vi "step6 Solve.vi"(8 "error in (no error)":errorcluster, 11 "cube in":T1) -> (0 "error out":errorcluster, 1 "all corners solved?":bool, 3 "cube out":T1)   [LabVIEW 2011]
doc: "Rotate cube as necessary so that the top middle piece matches the desired start colour.\n\nNo transformations are done in this VI, the operations are loaded on the the operation queue bus."
uses:
  Typedef/cube.ctl
  Typedef/face.ctl
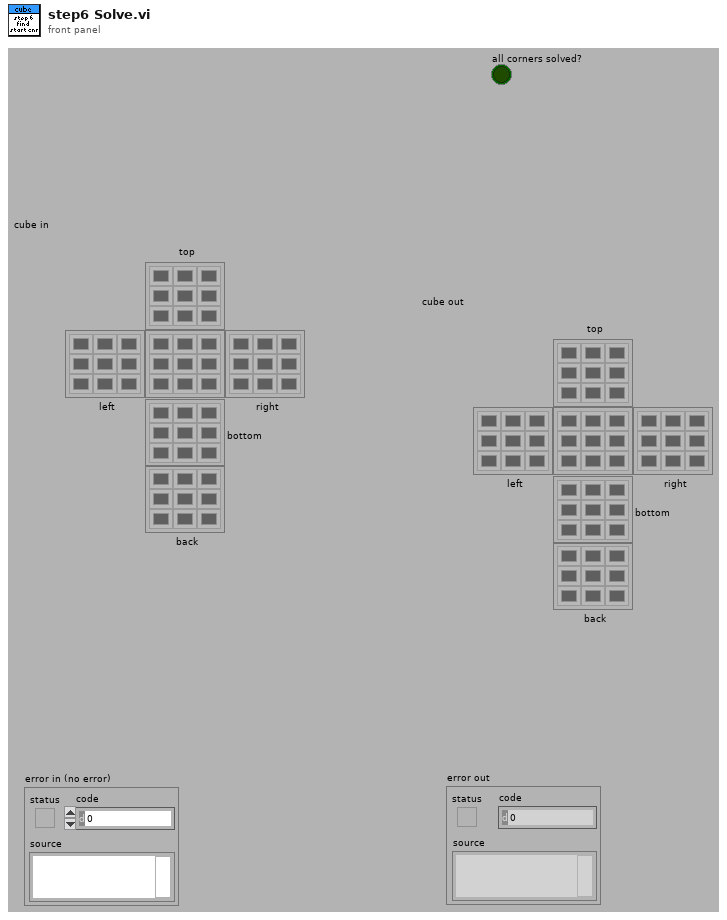
[diagram p1: front panel]
types:
  T1 = typedef "cube.ctl" = cluster{"top":T2, "left":T2, "right":T2, "bottom":T2, "back":T2, "front":T2}
  T2 = typedef "face.ctl" = u32[][]
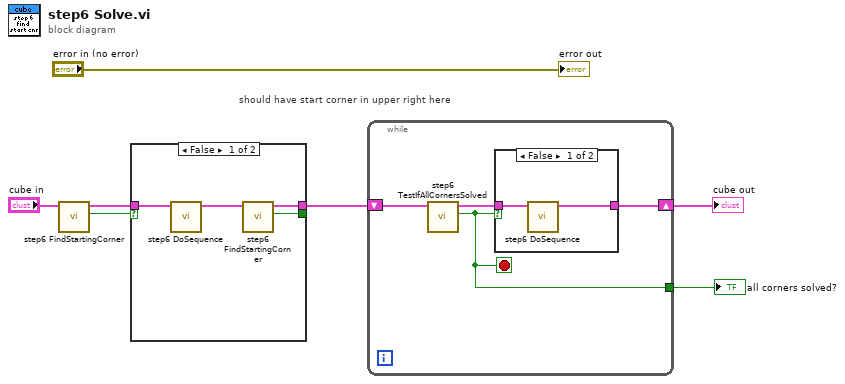
[diagram p0: block diagram]
diagram:
  # "should have start corner in upper right here"
  n1 = call "step6 FindStartingCorner.vi"("cube in"="cube in") -> ("found start corner?"=w5:bool, "cube out"=w4:T1)  [unwired: 9 in]
  n2 = case shown="False" w5 {
    tunnel: w4 -> [w11 w12]
    tunnel: [w9 w12] -> w3
    tunnel: [w8 _] -> _
    frame False {
      n3 = call "step6 DoSequence.vi"("cube in"=w11) -> ("cube out"=w10:T1)  [unwired: 10 in]
      n4 = call "step6 FindStartingCorner.vi"("cube in"=w10) -> ("found start corner?"=w8:bool, "cube out"=w9:T1)  [unwired: 9 in]
    }
    frame True {
    }
  }
  n5 = while {
    shift-right: [w14] -> w2
    shift-left: w3 -> [w16]
    tunnel: [w13] -> w1
    stop <- w13 stop-if-true
    n6 = call "step6 TestIfAllCornersSolved.vi"("cube in 2"=w16) -> ("all corners solved?"=w13:bool, "cube in"=w15:T1)  [unwired: 9 in]
    n7 = case shown="False" w13 {
      tunnel: w15 -> [w18 w19]
      tunnel: [w17 w19] -> w14
      frame False {
        n8 = call "step6 DoSequence.vi"("cube in"=w18) -> ("cube out"=w17:T1)  [unwired: 10 in]
      }
      frame True {
      }
    }
  }
  "cube out" <- w2
  "all corners solved?" <- w1
  "error out" <- "error in (no error)"
